vi "Set Remove Device Event.vi"(8 "error in (no error)":errorcluster, 10 "Remove Device":refnum<user-event>, 11 "DeviceDetailPanel in":refnum<class "DeviceDetailPanel.lvclass">) -> (0 "error out":errorcluster, 3 "DeviceDetailPanel out":refnum<class "DeviceDetailPanel.lvclass">)   [LabVIEW 2020, in "PicoG-App.lvlib" / "DeviceDetailPanel.lvclass"]
uses:
  DeviceDetailPanel.lvclass
  Device/Device.lvclass
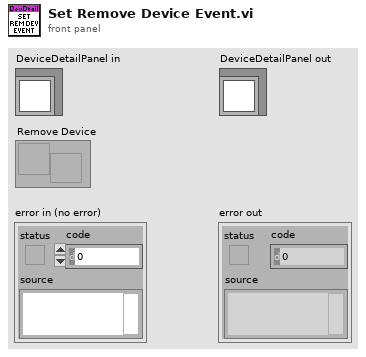
[diagram p1: front panel]
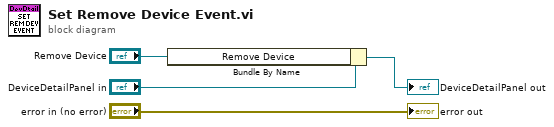
[diagram p0: block diagram]
diagram:
  n1 = Bundle By Name(cluster="DeviceDetailPanel in", "Remove Device"="Remove Device") -> (→"DeviceDetailPanel out":refnum<class "DeviceDetailPanel.lvclass">)
  "error out" <- "error in (no error)"
